vi "QrCodeBuild0.vi"(2 "有边缘？":bool=TRUE, 3 "ErrorCorrectLevel":i32(ring) items=["L", "M", "Q", "H"], 4 "Scale":u8=4, 5 "Text":string="HZHEHUA") -> (1 "out Array":bool[][](array[boolean]))   [LabVIEW 2018]
uses:
  Gma.QrCodeNet.Encoding.dll
panel:
  in  "停止":bool
  in  "QrCodeImgControl":refnum<k24>(container)
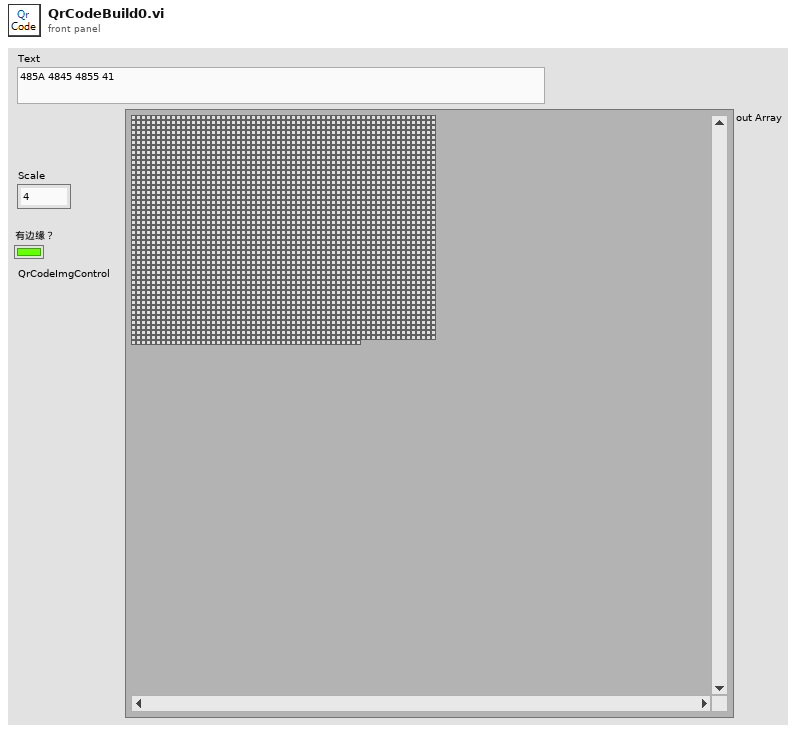
[diagram p1: front panel]
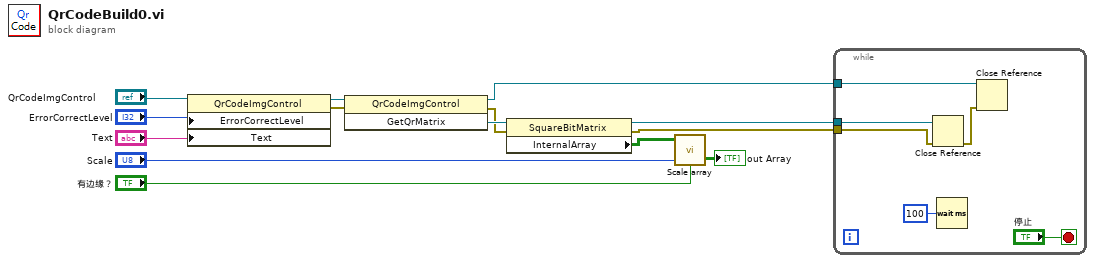
[diagram p0: block diagram]
diagram:
  n1 = property class="QrCodeImgControl"(reference="QrCodeImgControl", "ErrorCorrectLevel"="ErrorCorrectLevel", "Text"="Text") -> (reference out=w2:refnum<k24>, error out=w8:errorcluster)  [unwired: 1 in]
  n2 = invoke class="QrCodeImgControl" method="GetQrMatrix"(reference=w2, error in=w8) -> (reference out=w5:refnum<k24>, error out=w6:errorcluster, "GetQrMatrix"=w7:refnum<k24>)  [unwired: 1 in]
  n3 = property class="SquareBitMatrix"(reference=w7, error in=w6) -> (reference out=w4:refnum<k24>, error out=w1:errorcluster, "InternalArray"=w3:bool[][])
  n4 = call "Scale array.vi"("有边缘？"="有边缘？", "Scale"="Scale", "in Array"=w3) -> ("out Array"=→"out Array":bool[][])  [unwired: 1 in, 1 out]
  n5 = while {
    tunnel: w5 -> [w20]
    tunnel: w4 -> [w19]
    tunnel: w1 -> [w18]
    stop <- "停止" stop-if-true
    n6 = Close Reference(reference=w19, error in (no error)=w18) -> (error out=w17:errorcluster)
    n7 = Wait (ms)(milliseconds to wait=u32 100 ("等待时间（毫秒）")) -> ()  [unwired: 1 out]
    n8 = Close Reference(reference=w20, error in (no error)=w17) -> ()  [unwired: 1 out]
  }
